vi "sub_read_avi.vi"() -> (0 "Frames Per Second":u32, 1 "image array":T1[](array[typedef]))   [LabVIEW 2014]
uses:
  <vilib>/vision/Image Controls.llb/IMAQ Image.ctl
panel:
  in  "Stop":bool
  out "Progress Bar":i32(slide) max=135 scale=1.0..135.0
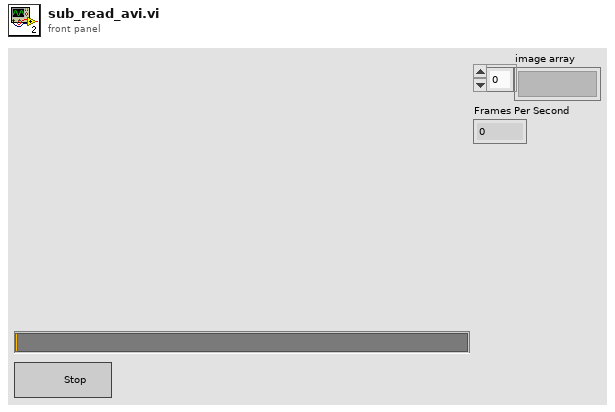
[diagram p1: front panel]
types:
  T1 = typedef "IMAQ Image.ctl" = refnum<image>
  T2 = typedef "IMAQ AVI2 Refnum.ctl" = refnum<k20>
  T3 = typedef "Image Type" = u32
  T4 = cluster{"Width":u32, "Height":u32, "Frames Per Second":u32, "Codec":string, "Has Data":bool}
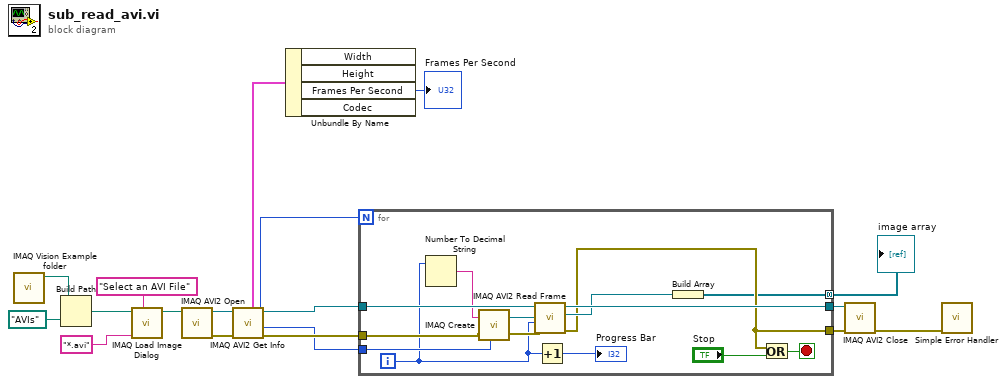
[diagram p0: block diagram]
diagram:
  n1 = call "IMAQ Vision Example folder.vi"() -> ("Example Image Path"=w13:path)  [unwired: 11 in]
  n2 = Build Path(base path=w13, name or relative path=path "AVIs") -> (appended path=w10:path)
  n3 = call "IMAQ Load Image Dialog"("Prompt"="Select an AVI File" ("prompt"), "Pattern"="*.avi", "Start Path"=w10) -> ("Path"=w9:path)  [unwired: 6 in, 2 out]
  n4 = call "IMAQ AVI2 Open"("AVI File Path"=w9) -> ("error out"=w18:errorcluster, "AVI Refnum"=w17:T2)  [unwired: 2 in, 7 out]
  n5 = call "IMAQ AVI2 Get Info"("error in (no error)"=w18, "AVI Refnum"=w17) -> ("error out"=w3:errorcluster, "Image Type"=w2:T3, "Number of Frames"=w1:u32, "AVI Refnum (duplicate)"=w14:T2, "Frame Data"=w5:T4)  [unwired: 5 out]
  n6 = Unbundle By Name(w5) -> ("Frames Per Second"=→"Frames Per Second":u32)  [unwired: 3 out]
  n7 = for {
    N: w1 -> [_]
    tunnel: [w31] -> w15
    tunnel: [w26] -> w16
    tunnel: w14 -> [w32]
    tunnel: [w25] -> w6 mode=concatenating
    tunnel: w3 -> [w22]
    tunnel: w2 -> [w21]
    i -> [w20]
    stop <- w28 stop-if-true
    n8 = Number To Decimal String(number=w20) -> (decimal integer string=w19:string)  [unwired: 1 in]
    n9 = call "IMAQ Create"("Image Name"=w19, "Image Type"=w21, "error in (no error)"=w22) -> ("New Image"=w24:T1, "error out"=w23:errorcluster)  [unwired: 1 in, 1 out]
    n10 = call "IMAQ AVI2 Read Frame"("error in (no error)"=w23, "Frame Number"=w20, "Image"=w24, "AVI Refnum"=w32) -> ("error out"=w26:errorcluster, "Image Out"=w30:T1, "AVI Refnum (duplicate)"=w31:T2)  [unwired: 5 out]
    n11 = Increment(x=w20) -> (x+1=→"Progress Bar":i32)
    n12 = Build Array(w30) -> (w25:T1[])
    n13 = Or(x=w26, y="Stop") -> (x .or. y?=w28:bool)
  }
  "image array" <- w6
  n14 = call "IMAQ AVI2 Close"("error in (no error)"=w16, "AVI Refnum"=w15) -> ("error out"=w7:errorcluster)  [unwired: 9 out]
  n15 = call <vilib>:"Simple Error Handler.vi"("error in (no error)"=w7) -> ()  [unwired: 1 in, 8 out]
